vi "Delete ChildPanel.vi"(8 "error in":errorcluster caption="错误输入（无错误）", 9 "Abort VI":bool, 10 "ChildNode*":refnum<data-value>, 11 "ParentNode in":refnum<class "PanelDataNode.lvclass"> caption="DNL_LabVIEW Object in") -> (0 "error out":errorcluster caption="错误输出", 2 "AnotherChildNode*":refnum<data-value>, 3 "Parent out":refnum<class "PanelDataNode.lvclass"> caption="DNL_LabVIEW Object out")   [LabVIEW 2016, in "PanelDataNode.lvclass"]
uses:
  PanelDataNode.lvclass
  C:/Users/CL/Desktop/ZcDAQprj0811/ZcDAQprj/Modules/DAQ-Display/PanelSplitToolkit/PanelLinkNode/PanelLinkNode.lvclass
  PanelObject/PanelObject.lvclass
  PanelLinkNode/PanelLinkNode.lvclass/PanelLinkNode.ctl
  PanelLinkNode/PanelLinkNode.lvclass
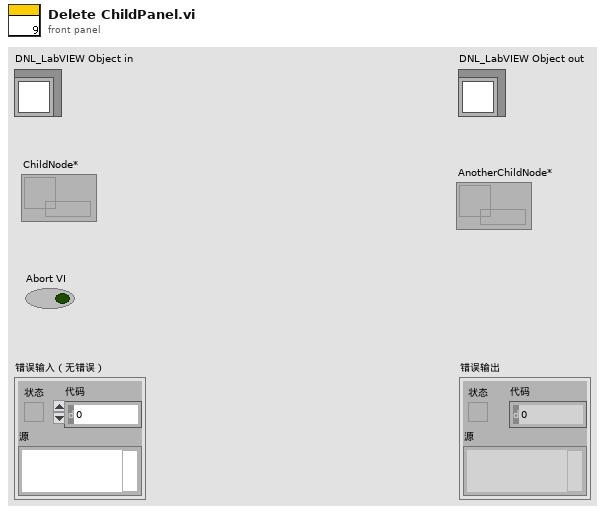
[diagram p1: front panel]
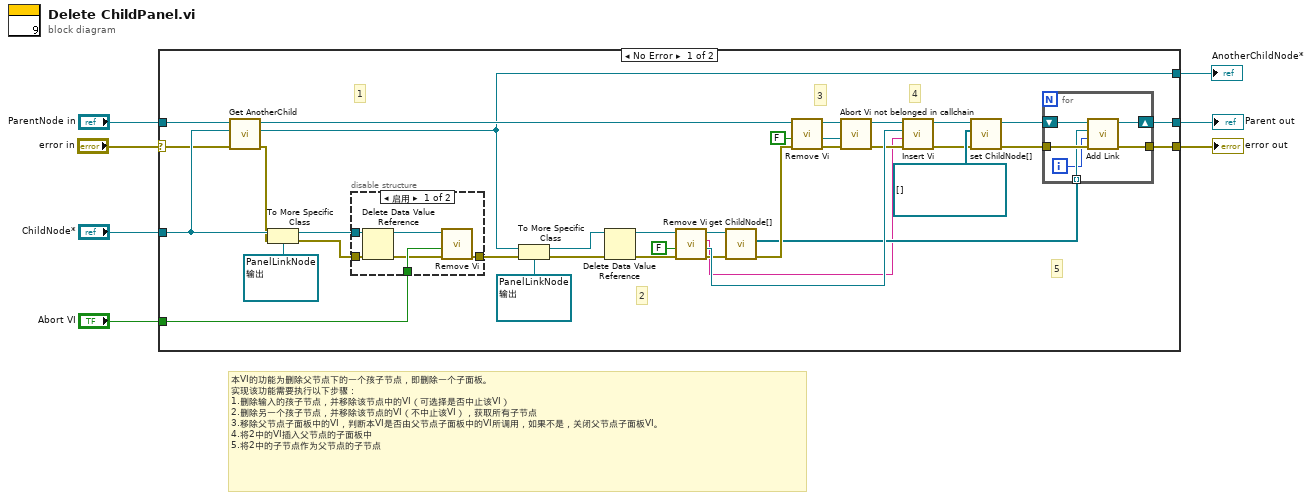
[diagram p0: block diagram]
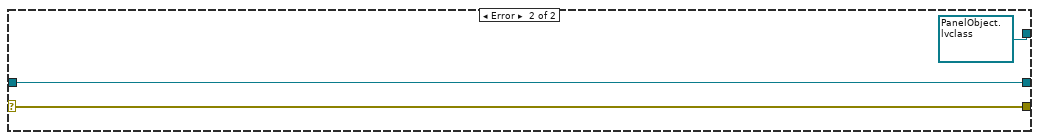
[diagram p3: hidden frame]
diagram:
  # "本VI的功能为删除父节点下的一个孩子节点，即删除一个子面板。\n实现该功能需要执行以下步骤：\n1.删除输入的孩子节点，并移除该节点中的VI（可选择是否中止该VI）\n2.删除另一个孩子节点，并移除该节点的VI（不中止该VI），获取所有子节点\n3.移除父节点子面板中的VI，判断本VI是否由父节点子面板中的VI所调用，如果不是，关闭父节点子面板VI。\n4.将2中的VI插入父节点的子面板中\n5.将2中的子节点作为父节点的子节点"
  n1 = case shown="No Error" "error in" {
    selector: "error in" -> [w21 w58]
    tunnel: [w16 w58] -> w6
    tunnel: [w18 w57] -> w4
    tunnel: "ParentNode in" -> [w41 w57]
    tunnel: "ChildNode*" -> [w26 _]
    tunnel: "Abort VI" -> [w42 _]
    tunnel: [w8 refnum<data-value> refnum ("AnotherChildNode*")] -> w1
    frame No Error {
      # "5"
      # "4"
      # "3"
      # "2"
      # "1"
      n2 = call-dynamic "Get AnotherChild.vi"("error in (no error)"=w21, "ChildNode*"=w26, "PanelLinkNode 输入"=w41) -> ("error out"=w14:errorcluster, "AnotherChildNode*"=w8:refnum<data-value>, "PanelLinkNode 输出"=w27:refnum<class "PanelDataNode.lvclass">)  [unwired: 6 in]
      n3 = To More Specific Class(target class=refnum<data-value> refnum ("数据值引用"), reference=w26, error in=w14) -> (specific class reference=w23:refnum<data-value>, error out=w13:errorcluster)
      n4 = disable-structure shown="启用" {
        disable-tunnel: w42 -> [w48 _]
        disable-tunnel: [w47 w49] -> w38
        disable-tunnel: w23 -> [w46 _]
        disable-tunnel: w13 -> [w45 w49]
        frame Enabled {
          n5 = Delete Data Value Reference(data value reference=w46, error in=w45) -> (data value=w43:refnum<class "PanelDataNode.lvclass">, error out=w44:errorcluster)
          n6 = call-dynamic "Remove Vi.vi"("error in"=w44, "Abort VI"=w48, "PanelDataNode 输入"=w43) -> ("error out"=w47:errorcluster)  [unwired: 5 in, 3 out]
        }
        frame Disabled {
        }
      }
      n7 = To More Specific Class(target class=refnum<data-value> refnum ("数据值引用"), reference=w8, error in=w38) -> (specific class reference=w39:refnum<data-value>, error out=w37:errorcluster)
      n8 = Delete Data Value Reference(data value reference=w39, error in=w37) -> (data value=w31:refnum<class "PanelDataNode.lvclass">, error out=w33:errorcluster)
      n9 = call-dynamic "Remove Vi.vi"("error in"=w33, "Abort VI"=FALSE, "PanelDataNode 输入"=w31) -> ("error out"=w32:errorcluster, "VI*"=w34:refnum<vi>, "ViValue"=w9:string, "PanelDataNode 输出"=w30:refnum<class "PanelDataNode.lvclass">)  [unwired: 5 in]
      n10 = call "get ChildNode[].vi"("error in (no error)"=w32, "PanelLinkNode输入"=w30) -> ("error out"=w29:errorcluster, "ChildNode*[]"=w15:refnum<data-value>[])  [unwired: 7 in, 1 out]
      n11 = call-dynamic "Remove Vi.vi"("error in"=w29, "Abort VI"=FALSE, "PanelDataNode 输入"=w27) -> ("error out"=w12:errorcluster, "VI*"=w25:refnum<vi>, "PanelDataNode 输出"=w35:refnum<class "PanelDataNode.lvclass">)  [unwired: 5 in, 1 out]
      n12 = call "Abort Vi not belonged in callchain.vi"("VI*"=w25, "error in (no error)"=w12) -> ("error out"=w11:errorcluster)  [unwired: 8 in]
      n13 = call-dynamic "Insert Vi.vi"("error in (no error)"=w11, "ViValue"=w9, "VI*"=w34, "PanelDataNode 输入"=w35) -> ("error out"=w10:errorcluster, "PanelDataNode 输出"=w36:refnum<class "PanelDataNode.lvclass">)  [unwired: 6 in]
      n14 = call "set ChildNode[].vi"("error in (no error)"=w10, "ChildNode*[]"=refnum<data-value>[] [], "PanelLinkNode输入"=w36) -> ("error out"=w17:errorcluster, "PanelLinkNode输出"=w19:refnum<class "PanelDataNode.lvclass">)  [unwired: 7 in]
      n15 = for {
        tunnel: w17 -> [w53]
        tunnel: [w52] -> w16
        tunnel: w15 -> [w51] mode=indexing
        shift-right: [w54] -> w18
        shift-left: w19 -> [w55]
        i -> [w50]
        n16 = call-dynamic "Add Link.vi"("ParentLinkNode in"=w55, "ChildNode* in"=w51, "L\\R Child"=w50, "error in (no error)"=w53) -> ("ParentLinkNode out"=w54:refnum<class "PanelDataNode.lvclass">, "error out"=w52:errorcluster)  [unwired: 5 in]
      }
    }
    frame Error {
    }
  }
  "error out" <- w6
  "Parent out" <- w4
  "AnotherChildNode*" <- w1
